vi "Global display 3.vi"() -> ()   [LabVIEW 2017]
panel:
  out "network drive":bool
  out "Ref deg C":dbl
  out "Amps Fail":dbl
  out "TEMP RS 05-2":cluster{"TL":dbl, "TN":dbl}
  out "TEMP ST 05-2":cluster{"TL":dbl, "TN":dbl}
  out "TEMP RS 05-1":cluster{"TL":dbl, "TN":dbl}
  out "TEMP ST 05-1":cluster{"TL":dbl, "TN":dbl}
  out "TEMP RS 04-2":cluster{"TL":dbl, "TN":dbl}
  out "TEMP ST 04-2":cluster{"TL":dbl, "TN":dbl}
  out "TEMP RS 04-1":cluster{"TL":dbl, "TN":dbl}
  out "TEMP ST 04-1":cluster{"TL":dbl, "TN":dbl}
  out "TEMP RS 03-2":cluster{"TL":dbl, "TN":dbl}
  out "TEMP ST 03-2":cluster{"TL":dbl, "TN":dbl}
  out "TEMP RS 03-1":cluster{"TL":dbl, "TN":dbl}
  out "TEMP ST 03-1":cluster{"TL":dbl, "TN":dbl}
  out "TEMP RS 02-2":cluster{"TL":dbl, "TN":dbl}
  out "TEMP ST 02-2":cluster{"TL":dbl, "TN":dbl}
  out "TEMP RS 02-1":cluster{"TL":dbl, "TN":dbl}
  out "TEMP ST 02-1":cluster{"TL":dbl, "TN":dbl}
  out "TEMP RS 01-2":cluster{"TL":dbl, "TN":dbl}
  out "TEMP ST 01-2":cluster{"TL":dbl, "TN":dbl}
  out "TEMP RS 01-1":cluster{"TL":dbl, "TN":dbl}
  out "TEMP ST 01-1":cluster{"TL":dbl, "TN":dbl}
  out "cycle O/F":bool
  out "graph deg C":dynamicdata(graph)
  out "graph volts":dynamicdata(graph)
  out "graph amps":dynamicdata(graph)
  out "admin":bool
  out "graph flag":bool
  out "log all":string
  out "log 5-2":string
  out "log 5-1":string
  out "log 4-2":string
  out "log 4-1":string
  out "log 3-2":string
  out "log 3-1":string
  out "log 2-2":string
  out "log 2-1":string
  out "log 1-2":string
  out "log 1-1":string
  out "CYCLE 5-2":dbl
  out "CYCLE 5-1":dbl
  out "CYCLE 4-2":dbl
  out "CYCLE 4-1":dbl
  out "CYCLE 3-2":dbl
  out "CYCLE 3-1":dbl
  out "CYCLE 2-2":dbl
  out "CYCLE 2-1":dbl
  out "CYCLE 1-2":dbl
  out "CYCLE 1-1":dbl
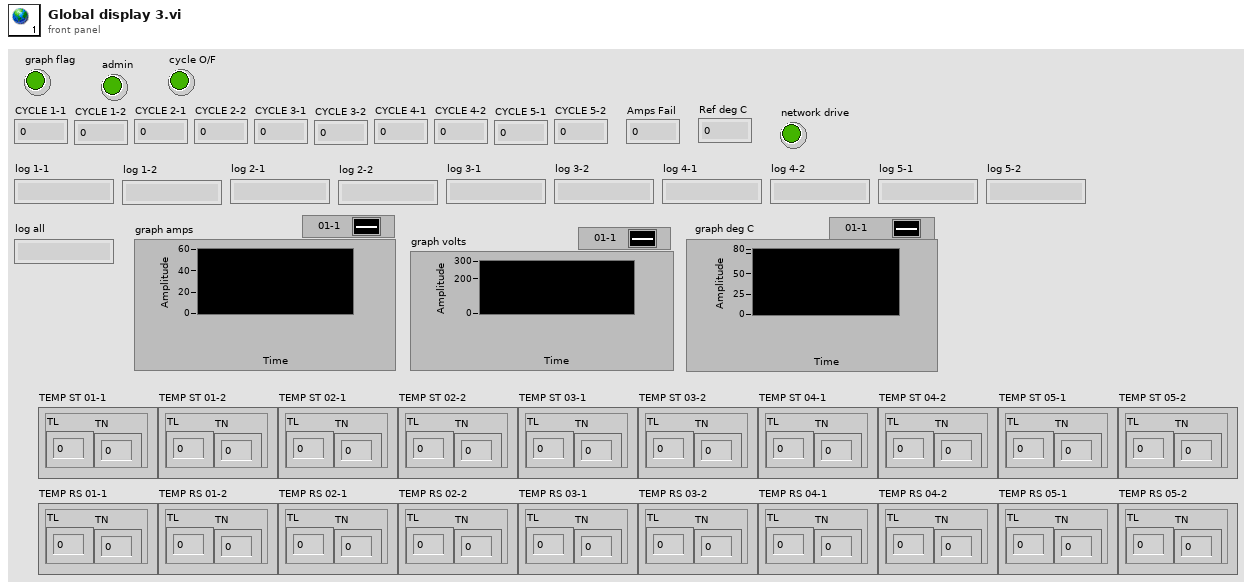
[diagram p1: front panel]
diagram:
